vi "String to KVP.vi"(8 "error in (no error)":errorcluster, 10 "Input String":string, 11 "ConfigManager.Text in":refnum<class "ConfigManager.Text.lvclass">) -> (0 "error out":errorcluster, 1 "Values":string[](array[string]), 2 "Keys":string[](array[string]), 3 "ConfigManager.Text out":refnum<class "ConfigManager.Text.lvclass">, 5 "Qualified Names":string[](array[string]))   [LabVIEW 2013, in "CfgManager.Text.lvlib" / "ConfigManager.Text.lvclass"]
uses:
  ConfigManager.Text.lvclass
  ConfigManager.Text.lvclass/ConfigManager.Text.ctl
  <vilib>/LabVIEW Open Source Project/Unicity/Delimiter/Delimiter.lvclass
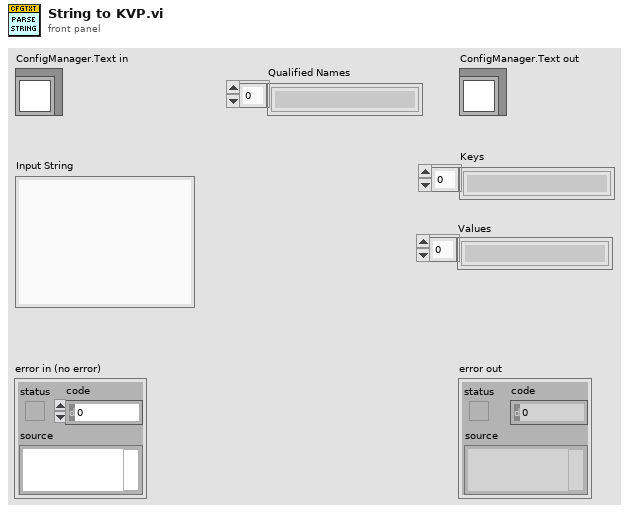
[diagram p1: front panel]
types:
  T1 = typedef "CfgManager.Text.lvlib/ConfigManager.Text.lvclass/Configuration -- Cluster.ctl" = cluster{"FileHeader":refnum<class "FileHeader.lvclass">, "FileSignature":refnum<class "FileSignature.lvclass">, "Section Delimiter":refnum<class "Delimiter.lvclass">, "Key-Value Separator":refnum<class "Delimiter.lvclass">}
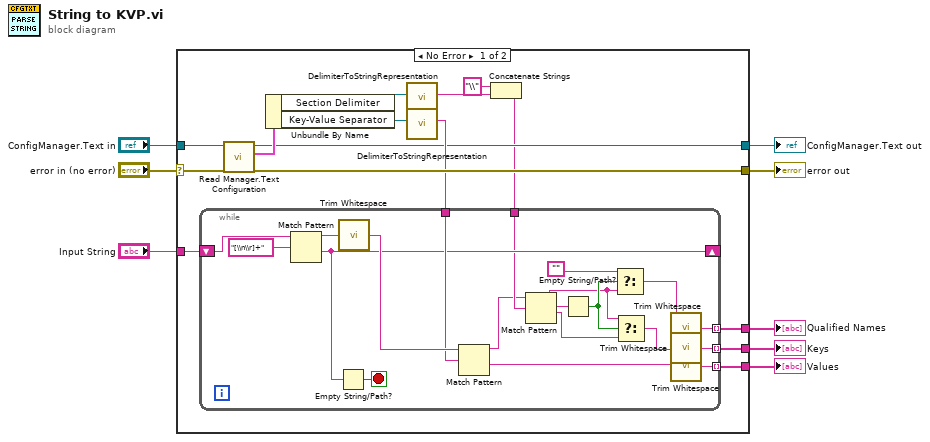
[diagram p0: block diagram]
diagram:
  n1 = case shown="No Error" "error in (no error)" {
    selector: "error in (no error)" -> [w22 w44]
    tunnel: [w22 w44] -> w7
    tunnel: [w14 w43] -> w5
    tunnel: "ConfigManager.Text in" -> [w19 w43]
    tunnel: "Input String" -> [w21 _]
    tunnel: [w20 _] -> w3
    tunnel: [w16 _] -> w2
    tunnel: [w13 _] -> w1
    frame No Error {
      n2 = call "Read Manager.Text Configuration.vi"("ConfigManager.Text in"=w19) -> ("Manager.Text Configuration"=w18:T1, "ConfigManager.Text out"=w14:refnum<class "ConfigManager.Text.lvclass">)  [unwired: 9 in]
      n3 = Unbundle By Name(w18) -> ("Section Delimiter"=w12:refnum<class "Delimiter.lvclass">, "Key-Value Separator"=w17:refnum<class "Delimiter.lvclass">)
      n4 = call <vilib>:"DelimiterToStringRepresentation.vi"("Delimiter"=w12) -> ("String representation"=w11:string)  [unwired: 10 in]
      n5 = call <vilib>:"DelimiterToStringRepresentation.vi"("Delimiter"=w17) -> ("String representation"=w15:string)  [unwired: 10 in]
      n6 = Concatenate Strings("\\" ("string"), w11) -> (w9:string)
      n7 = while {
        shift-right: [w34] -> _
        shift-left: w21 -> [w41]
        tunnel: [w37] -> w20 mode=indexing
        tunnel: w15 -> [w35]
        tunnel: [w33] -> w16 mode=indexing
        tunnel: [w28] -> w13 mode=indexing
        tunnel: w9 -> [w32]
        stop <- w42 stop-if-true
        n8 = Match Pattern(string=w41, regular expression="[\\n\\r]+") -> (before substring=w40:string, after substring=w34:string)  [unwired: 1 in, 2 out]
        n9 = Empty String/Path?(string/path=w34) -> (empty?=w42:bool)
        n10 = call <vilib>:"Trim Whitespace.vi"("string"=w40) -> ("trimmed string"=w38:string)  [unwired: 1 in]
        n11 = Match Pattern(string=w38, regular expression=w35) -> (before substring=w24:string, after substring=w36:string)  [unwired: 1 in, 2 out]
        n12 = Match Pattern(string=w24, regular expression=w32) -> (before substring=w26:string, match substring=w31:string, after substring=w25:string)  [unwired: 1 in, 1 out]
        n13 = Empty String/Path?(string/path=w31) -> (empty?=w29:bool)
        n14 = Select(t="", s=w29, f=w26) -> (s? t:f=w27:string)
        n15 = Select(t=w26, s=w29, f=w25) -> (s? t:f=w23:string)
        n16 = call <vilib>:"Trim Whitespace.vi"("string"=w27) -> ("trimmed string"=w28:string)  [unwired: 1 in]
        n17 = call <vilib>:"Trim Whitespace.vi"("string"=w23) -> ("trimmed string"=w37:string)  [unwired: 1 in]
        n18 = call <vilib>:"Trim Whitespace.vi"("string"=w36) -> ("trimmed string"=w33:string)  [unwired: 1 in]
      }
    }
    frame Error {
    }
  }
  "error out" <- w7
  "ConfigManager.Text out" <- w5
  "Keys" <- w3
  "Values" <- w2
  "Qualified Names" <- w1
